vi "Create Table.vi"(0 "PDF Report":T26(xcontrol), 1 "Table properties":T4={"Table position"=1, "SpacingBefore (points)"=12.0, "SpacingAfter (points)"=12.0} {"Table position" items=["LEFT", "CENTER", "RIGHT"]}, 3 "Title 1D":string[](array[string]), 7 "columnWidth [ ]":sgl[](array[numeric]), 11 "error in (no error)":errorcluster, 12 "Image to Add [ ]":T2 {"Scale" format="%#_g %"}, 14 "Table Datas 2D":string[][](array[string])) -> (4 "PDF Report duplicate":T26(xcontrol), 8 "PDF Table":T1(xcontrol), 15 "error out":errorcluster)   [LabVIEW 2012]
doc: "<B>ENGLISH</B>\n\nCreate a table (a cell can contain either text or an image, but not both).\n\n\n<B>1) Table 2D Datas</B> (<B>required</B>) \n2D text array.\n\n<B>2) Title 1D</B> (optional)\n1D text array.\n\n<B>3) Table Properties</B> (optional)\nPosition (left, center or right), spacing before and after.\n\n<B>4) columnWidht [ ]</B> (optional).\nWidth of each column.\n\n<B>5) Image to Add [ ]</B> (optional)\n\n<B>FRANÇAIS</B>\n\nCréation d'un tableau (une cellule peut contenir soit du texte ou soit une image mas pas les deux). \n\nDeveloped by Jean-Marc Simard\nCopyright © 2010, Exaprom Inc.\nAll rights reserved.\nLicense: BSD\n\nWith iTextSharp 4.1.6 (http://itextsharp.sourceforge.net)\nunder Mozilla Public License Version 1.1\n(http://www.mozilla.org/MPL/MPL-1.1.html)"
uses:
  Controls/PDF Report Xcontrol/PDF Report.xctl
  Controls/Table properties.ctl
  Controls/Table position.ctl
  Controls/Image to Add [ ].ctl
  Controls/Image Scale.ctl
  Controls/PDF Table Xcontrol/PDF Table XControl.xctl
  C:/Users/MaxCorp/Documents/TopPerm - Base/DLL/itextsharp.dll
  DLL/itextsharp.dll
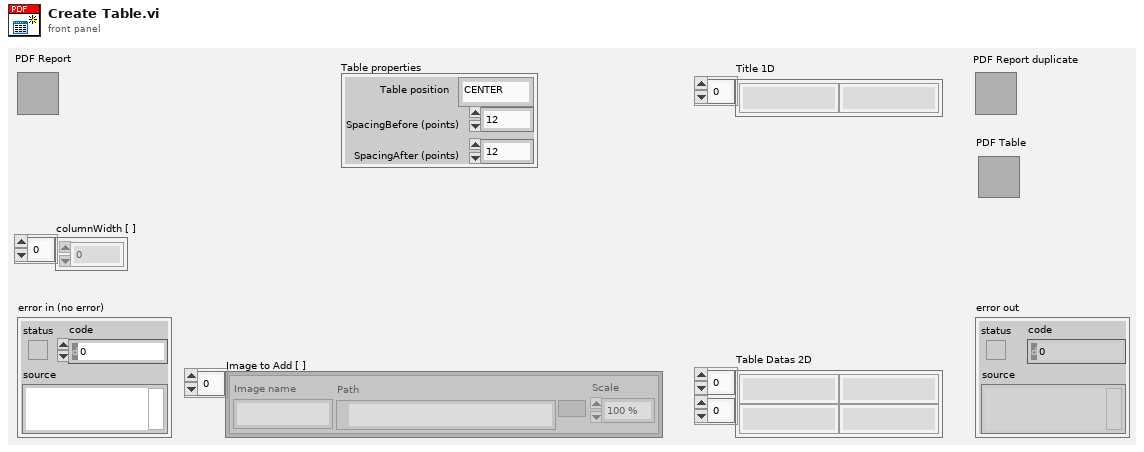
[diagram p1: front panel]
types:
  T1 = cluster{"PDFTable ref":refnum<k24>, "columnWidth (points)":sgl[], "Title 1D":string[], "Table Datas 2D":string[][], "Image to Add with refnum[ ]":cluster{"Image name":string, "InstanceImage":refnum<k24>}[]}
  T2 = typedef "Image to Add [ ].ctl" = cluster{"Image name":string, "Path":path, "Scale":T3}[]
  T3 = typedef "Image Scale.ctl" = sgl
  T4 = typedef "Table properties.ctl" = cluster{"Table position":T5, "SpacingBefore (points)":sgl, "SpacingAfter (points)":sgl}
  T5 = typedef "Table position.ctl" = i32
  T6 = typedef "Font cluster.ctl" = cluster{"Name":string, "Size":T7, "Color":T8, "Style":cluster{"Bold":bool, "Italic":bool, "Underline":bool, "Strikeout":bool}}
  T7 = typedef "Font size.ctl" = sgl
  T8 = typedef "Font color.ctl" = u32
  T9 = typedef "Unit.ctl" = enum16{"inch", "mm"}
  T10 = typedef "Paragraphe cluster.ctl" = cluster{" Aligment":T11, "Line spacing":T12}
  T11 = typedef "Texte alignement.ctl" = enum16{"Select", "CENTER", "JUSTIFY", "LEFT", "RIGHT"}
  T12 = typedef "Line spacing.ctl" = enum16{"Select", "1.0", "1.5", "2.0"}
  T13 = typedef "Page dimensions.ctl" = cluster{"Start at page":i32, "Orientation":T14, "widht":sgl, "height":sgl, "Margin left":sgl, "Margin right":sgl, "Margin top":sgl, "Margin bottom":sgl}
  T14 = typedef "Page Orientation.ctl" = enum16{"Portrait", "Landscape"}
  T15 = typedef "Image or Table Caption.ctl" = cluster{"Caption":string, "Separator":string, "Position":enum16{"Above", "Below"}}
  T16 = typedef "Header Footer [ ].ctl" = T17[]
  T17 = typedef "Header Footer cluster.ctl" = cluster{"Start page":i32, "Type":T18, "Alignment":T19, "Vertical Alignement":T20, "Image (%)":sgl, "Page #":T21, "Text":string, "Path":string, "Font":T6, "Font refnum":refnum<k24>, "Line":cluster{"Line":T22, "Thickness (points)":sgl, "Colour":T8}}
  T18 = typedef "Header Footer Type.ctl" = enum16{"Select", "Text", "Text + hyperlink", "Page number", "Image", "Image + hyperlink"}
  T19 = typedef "Header footer horiz alignment.ctl" = enum16{"Left", "Center", "Right"}
  T20 = typedef "Cell Vertical alignment.ctl" = enum16{"TOP", "MIDDLE", "BOTTOM"}
  T21 = typedef "Page number.ctl" = cluster{"Text 1":string, "Text 2":string, "Text 3":string}
  T22 = typedef "Header Footer Line.ctl" = enum16{"No line", "Horizontal line"}
  T23 = typedef "Watermark cluster2.ctl" = cluster{"Show? (F)":bool, "Type":enum16{"Image", "Text"}, "Opacity (%)":sgl, "Rotate(°)":sgl, "Position":cluster{"Position":T24, "X":sgl, "Y":sgl}, "Image path":path, "Scaled(%)":sgl, "Image refnum":refnum<k24>, "Text":string, "Font":cluster{"Name":string, "Size":T7, "Color":T8}, "Font refnum":refnum<k24>, "Alignment":T19, "Automatic":bool}
  T24 = typedef "Watermark Position.ctl" = enum16{"Absolute", "Center (page)", "Center (text section)"}
  T25 = typedef "System Fonts.ctl" = cluster{"Font name [ ]":string[], "Font and file names [ ]":cluster{"Font name":string, "File name":string}[]}
  T26 = cluster{"Document":refnum<k24>, "Writer":refnum<k24>, "Default Font":refnum<k24>, "Default Font cluster":T6, "Path":path, "Unit (default = mm)":T9, "Paragraphe cluster":T10, "Pages dimensions [ ]":T13[], "Captions":cluster{"Image":T15, "Image counter":u16, "Table":T15, "Table counter":u16, "Font":T6}, "Header":T16, "Footer":T16, "Watermark ":T23, "Actual VI name":string, "System Fonts":T25}
  T27 = typedef "Image to Add refnum [ ].ctl" = cluster{"Image name":string, "InstanceImage":refnum<k24>}[]
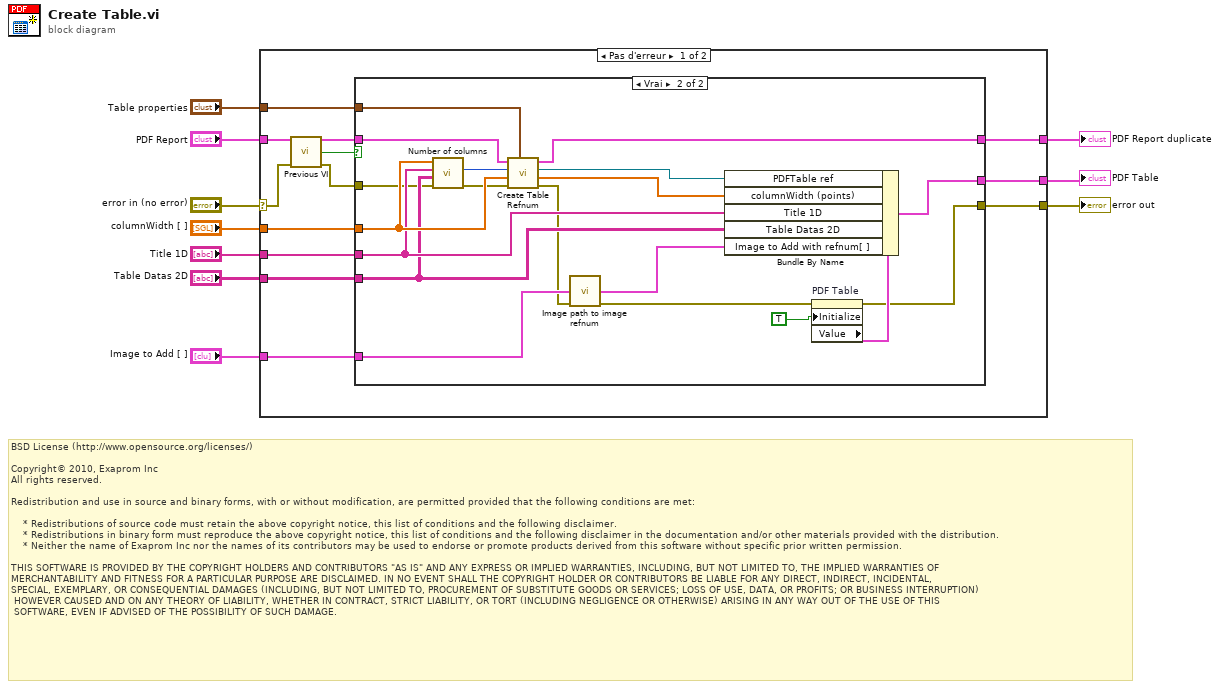
[diagram p0: block diagram]
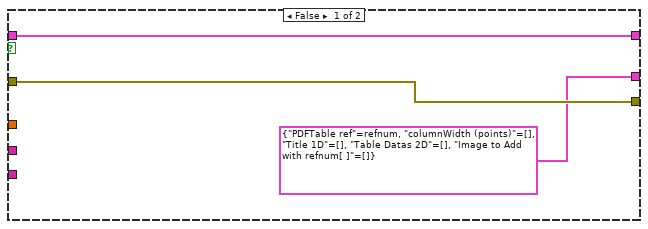
[diagram p2: hidden frame]
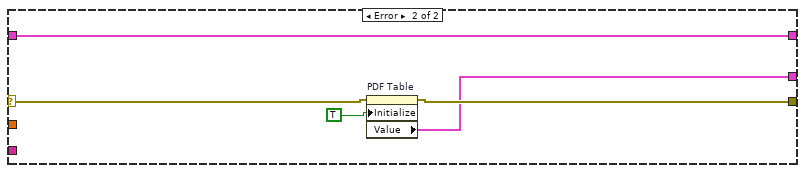
[diagram p3: hidden frame]
diagram:
  # "BSD License (http://www.opensource.org/licenses/)\n\nCopyright© 2010, Exaprom Inc\nAll rights reserved.\n\nRedistribution and use in source and binary forms, with or without modification, are permitted provided that the following conditions are met:\n\n    * Redistributions of source code must retain the above copyright notice, this list of conditions and the following disclaimer.\n    * Redistributions in binary form must reproduce the above copyright notice, this list of conditions and the following disclaimer in the documentation and/or other materials provided with the distribution.\n    * Neither the name of Exaprom Inc nor the names of its contributors may be used to endorse or promote products derived from this software without specific prior written permission.\n\nTHIS SOFTWARE IS PROVIDED BY THE COPYRIGHT HOLDERS AND CONTRIBUTORS \"AS IS\" AND ANY EXPRESS OR IMPLIED WARRANTIES, INCLUDING, BUT NOT LIMITED TO, THE IMPLIED WARRANTIES OF \nMERCHANTABILITY AND FITNESS FOR A PARTICULAR PURPOSE ARE DISCLAIMED. IN NO EVENT SHALL THE COPYRIGHT HOLDER OR CONTRIBUTORS BE LIABLE FOR ANY DIRECT, INDIRECT, INCIDENTAL,\nSPECIAL, EXEMPLARY, OR CONSEQUENTIAL DAMAGES (INCLUDING, BUT NOT LIMITED TO, PROCUREMENT OF SUBSTITUTE GOODS OR SERVICES; LOSS OF USE, DATA, OR PROFITS; OR BUSINESS INTERRUPTION)\n HOWEVER CAUSED AND ON ANY THEORY OF LIABILITY, WHETHER IN CONTRACT, STRICT LIABILITY, OR TORT (INCLUDING NEGLIGENCE OR OTHERWISE) ARISING IN ANY WAY OUT OF THE USE OF THIS\n SOFTWARE, EVEN IF ADVISED OF THE POSSIBILITY OF SUCH DAMAGE."
  n1 = case shown="Pas d'erreur" "error in (no error)" {
    selector: "error in (no error)" -> [w13 w49]
    tunnel: "columnWidth [ ]" -> [w19 _]
    tunnel: [w16 w48] -> w8
    tunnel: [w23 w50] -> w7
    tunnel: "PDF Report" -> [w21 w50]
    tunnel: "Table properties" -> [w22 _]
    tunnel: [w15 w46] -> w1
    tunnel: "Title 1D" -> [w18 _]
    tunnel: "Table Datas 2D" -> [w17 _]
    tunnel: "Image to Add [ ]" -> [w20 _]
    frame No Error {
      n2 = call "Previous VI.vi"("PDF Report IN"=w21, "error in (no error)"=w13) -> ("PDF Report OUT"=w14:T26, "Execute Actual VI"=w12:bool, "error out"=w11:errorcluster)  [unwired: 11 out]
      n3 = case shown="Vrai" w12 {
        tunnel: [w26 w45] -> w23
        tunnel: w22 -> [_ w44]
        tunnel: w20 -> [_ w41]
        tunnel: w19 -> [_ w40]
        tunnel: w18 -> [_ w39]
        tunnel: w17 -> [_ w38]
        tunnel: [w25 w32] -> w16
        tunnel: [T1 {"PDFTable ref"=refnum, "columnWidth (points)"=[], "Title 1D"=[], "Table Datas 2D"=[], "Image to Add with refnum[ ]"=[]} ("PDF Table") w30] -> w15
        tunnel: w14 -> [w26 w29]
        tunnel: w11 -> [w25 w28]
        frame False {
        }
        frame True {
          n4 = call "Number of columns.vi"("error in (no error)"=w28, "Table Datas 2D"=w38, "Title 1D"=w39, "columnWidth [ ]"=w40) -> ("error duplicate"=w27:errorcluster, "numColumns"=w37:i32)  [unwired: 6 out]
          n5 = call "Create Table Refnum.vi"("Table properties"=w44, "error in (no error)"=w27, "columnWidth [ ]"=w40, "numColumns"=w37, "PDF Report"=w29) -> ("error out"=w34:errorcluster, "columnWidth (points)"=w42:sgl[], "PdfP Table ref"=w43:refnum<k24>, "PDF Report duplicate"=w45:T26)  [unwired: 1 out]
          n6 = call "Image path to image refnum.vi"("Image to Add [ ]"=w41, "error in (no error)"=w34) -> ("Image to Add refnum [ ]"=w31:T27, "error out"=w33:errorcluster)  [unwired: 12 out]
          n7 = property on="PDF Table" class="PDF Table XControl (strict)"(error in=w33, "Initialize"=TRUE) -> (error out=w32:errorcluster, "Value"=w35:T1)  [unwired: 1 in, 1 out]
          n8 = Bundle By Name(cluster=w35, "PDFTable ref"=w43, "columnWidth (points)"=w42, "Title 1D"=w39, "Table Datas 2D"=w38, "Image to Add with refnum[ ]"=w31) -> (w30:T1)
        }
      }
    }
    frame Error {
      n9 = property on="PDF Table" class="PDF Table XControl (strict)"(error in=w49, "Initialize"=TRUE) -> (error out=w48:errorcluster, "Value"=w46:T1)  [unwired: 1 in, 1 out]
    }
  }
  "error out" <- w8
  "PDF Report duplicate" <- w7
  "PDF Table" <- w1
